vi "Big Boolean Cluster.vi"(1 "Cluster":T1) -> (0 "Cluster out":T1)   [LabVIEW 2010]
types:
  T1 = cluster{"Boolean":bool, "Boolean 2":bool, "Boolean 3":bool, "Boolean 4":bool, "Boolean 5":bool, "Boolean 6":bool, "Boolean 7":bool, "Boolean 8":bool, "Boolean 9":bool, "Boolean 10":bool, "Boolean 11":bool, "Boolean 12":bool, "Boolean 13":bool, "Boolean 14":bool, "Boolean 15":bool, "Boolean 16":bool, "Boolean 17":bool, "Boolean 18":bool, "Boolean 19":bool, "Boolean 20":bool, "Boolean 21":bool, "Boolean 22":bool, "Boolean 23":bool, "Boolean 24":bool, "Boolean 25":bool, "Boolean 26":bool, "Boolean 27":bool, "Boolean 28":bool, "Boolean 29":bool, "Boolean 30":bool, "Boolean 31":bool, "Boolean 32":bool, "Boolean 33":bool, "Boolean 34":bool, "Boolean 35":bool, "Boolean 36":bool, "Boolean 37":bool, "Boolean 38":bool, "Boolean 39":bool, "Boolean 40":bool, "Boolean 41":bool, "Boolean 42":bool, "Boolean 43":bool, "Boolean 44":bool, "Boolean 45":bool, "Boolean 46":bool, "Boolean 47":bool, "Boolean 48":bool, "Boolean 49":bool, "Boolean 50":bool, "Boolean 51":bool, "Boolean 52":bool, "Boolean 53":bool, "Boolean 54":bool, "Boolean 55":bool, "Boolean 56":bool, "Boolean 57":bool, "Boolean 58":bool, "Boolean 59":bool, "Boolean 60":bool, "Boolean 61":bool, "Boolean 62":bool, "Boolean 63":bool, "Boolean 64":bool, "Boolean 65":bool, "Boolean 66":bool, "Boolean 67":bool, "Boolean 68":bool, "Boolean 69":bool, "Boolean 70":bool, "Boolean 71":bool, "Boolean 72":bool, "Boolean 73":bool, "Boolean 74":bool, "Boolean 75":bool, "Boolean 76":bool, "Boolean 77":bool, "Boolean 78":bool, "Boolean 79":bool, "Boolean 80":bool, "Boolean 81":bool, "Boolean 82":bool, "Boolean 83":bool, "Boolean 84":bool, "Boolean 85":bool, "Boolean 86":bool, "Boolean 87":bool, "Boolean 88":bool, "Boolean 89":bool, "Boolean 90":bool, "Boolean 91":bool, "Boolean 92":bool, "Boolean 93":bool, "Boolean 94":bool, "Boolean 95":bool, "Boolean 96":bool, "Boolean 97":bool, "Boolean 98":bool, "Boolean 99":bool, "Boolean 100":bool, "Boolean 101":bool, "Boolean 102":bool, "Boolean 103":bool, "Boolean 104":bool, "Boolean 105":bool, "Boolean 106":bool, "Boolean 107":bool, "Boolean 108":bool, "Boolean 109":bool, "Boolean 110":bool, "Boolean 111":bool, "Boolean 112":bool, "Boolean 113":bool, "Boolean 114":bool, "Boolean 115":bool, "Boolean 116":bool, "Boolean 117":bool, "Boolean 118":bool, "Boolean 119":bool, "Boolean 120":bool, "Boolean 121":bool, "Boolean 122":bool, "Boolean 123":bool, "Boolean 124":bool, "Boolean 125":bool, "Boolean 126":bool, "Boolean 127":bool, "Boolean 128":bool, "Boolean 129":bool, "Boolean 130":bool, "Boolean 131":bool, "Boolean 132":bool, "Boolean 133":bool, "Boolean 134":bool, "Boolean 135":bool, "Boolean 136":bool, "Boolean 137":bool, "Boolean 138":bool, "Boolean 139":bool, "Boolean 140":bool, "Boolean 141":bool, "Boolean 142":bool, "Boolean 143":bool, "Boolean 144":bool, "Boolean 145":bool, "Boolean 146":bool, "Boolean 147":bool, "Boolean 148":bool, "Boolean 149":bool, "Boolean 150":bool, "Boolean 151":bool, "Boolean 152":bool, "Boolean 153":bool, "Boolean 154":bool, "Boolean 155":bool, "Boolean 156":bool, "Boolean 157":bool, "Boolean 158":bool, "Boolean 159":bool, "Boolean 160":bool, "Boolean 161":bool, "Boolean 162":bool, "Boolean 163":bool, "Boolean 164":bool, "Boolean 165":bool, "Boolean 166":bool, "Boolean 167":bool, "Boolean 168":bool, "Boolean 169":bool, "Boolean 170":bool, "Boolean 171":bool, "Boolean 172":bool, "Boolean 173":bool, "Boolean 174":bool, "Boolean 175":bool, "Boolean 176":bool, "Boolean 177":bool, "Boolean 178":bool, "Boolean 179":bool, "Boolean 180":bool, "Boolean 181":bool, "Boolean 182":bool, "Boolean 183":bool, "Boolean 184":bool, "Boolean 185":bool, "Boolean 186":bool, "Boolean 187":bool, "Boolean 188":bool, "Boolean 189":bool, "Boolean 190":bool, "Boolean 191":bool, "Boolean 192":bool, "Boolean 193":bool, "Boolean 194":bool, "Boolean 195":bool, "Boolean 196":bool, "Boolean 197":bool, "Boolean 198":bool, "Boolean 199":bool, "Boolean 200":bool, "Boolean 201":bool, "Boolean 202":bool, "Boolean 203":bool, "Boolean 204":bool, "Boolean 205":bool, "Boolean 206":bool, "Boolean 207":bool, "Boolean 208":bool, "Boolean 209":bool, "Boolean 210":bool, "Boolean 211":bool, "Boolean 212":bool, "Boolean 213":bool, "Boolean 214":bool, "Boolean 215":bool, "Boolean 216":bool, "Boolean 217":bool, "Boolean 218":bool, "Boolean 219":bool, "Boolean 220":bool, "Boolean 221":bool, "Boolean 222":bool, "Boolean 223":bool, "Boolean 224":bool, "Boolean 225":bool, "Boolean 226":bool, "Boolean 227":bool, "Boolean 228":bool, "Boolean 229":bool, "Boolean 230":bool, "Boolean 231":bool, "Boolean 232":bool, "Boolean 233":bool, "Boolean 234":bool, "Boolean 235":bool, "Boolean 236":bool, "Boolean 237":bool, "Boolean 238":bool, "Boolean 239":bool, "Boolean 240":bool, "Boolean 241":bool, "Boolean 242":bool, "Boolean 243":bool, "Boolean 244":bool, "Boolean 245":bool, "Boolean 246":bool, "Boolean 247":bool, "Boolean 248":bool, "Boolean 249":bool, "Boolean 250":bool, "Boolean 251":bool, "Boolean 252":bool, "Boolean 253":bool, "Boolean 254":bool, "Boolean 255":bool, "Boolean 256":bool, "Boolean 257":bool, "Boolean 258":bool, "Boolean 259":bool, "Boolean 260":bool, "Boolean 261":bool, "Boolean 262":bool, "Boolean 263":bool, "Boolean 264":bool, "Boolean 265":bool, "Boolean 266":bool, "Boolean 267":bool, "Boolean 268":bool, "Boolean 269":bool, "Boolean 270":bool, "Boolean 271":bool, "Boolean 272":bool, "Boolean 273":bool, "Boolean 274":bool, "Boolean 275":bool, "Boolean 276":bool, "Boolean 277":bool, "Boolean 278":bool, "Boolean 279":bool, "Boolean 280":bool, "Boolean 281":bool, "Boolean 282":bool, "Boolean 283":bool, "Boolean 284":bool, "Boolean 285":bool, "Boolean 286":bool, "Boolean 287":bool, "Boolean 288":bool, "Boolean 289":bool, "Boolean 290":bool, "Boolean 291":bool, "Boolean 292":bool, "Boolean 293":bool, "Boolean 294":bool, "Boolean 295":bool, "Boolean 296":bool, "Boolean 297":bool, "Boolean 298":bool, "Boolean 299":bool, "Boolean 300":bool, "Boolean 301":bool, "Boolean 302":bool, "Boolean 303":bool, "Boolean 304":bool, "Boolean 305":bool, "Boolean 306":bool, "Boolean 307":bool, "Boolean 308":bool, "Boolean 309":bool, "Boolean 310":bool, "Boolean 311":bool, "Boolean 312":bool, "Boolean 313":bool, "Boolean 314":bool, "Boolean 315":bool, "Boolean 316":bool, "Boolean 317":bool, "Boolean 318":bool, "Boolean 319":bool, "Boolean 320":bool, "Boolean 321":bool, "Boolean 322":bool, "Boolean 323":bool, "Boolean 324":bool, "Boolean 325":bool, "Boolean 326":bool, "Boolean 327":bool, "Boolean 328":bool, "Boolean 329":bool, "Boolean 330":bool, "Boolean 331":bool, "Boolean 332":bool, "Boolean 333":bool, "Boolean 334":bool, "Boolean 335":bool, "Boolean 336":bool, "Boolean 337":bool, "Boolean 338":bool, "Boolean 339":bool, "Boolean 340":bool, "Boolean 341":bool, "Boolean 342":bool, "Boolean 343":bool, "Boolean 344":bool, "Boolean 345":bool, "Boolean 346":bool, "Boolean 347":bool, "Boolean 348":bool, "Boolean 349":bool, "Boolean 350":bool, "Boolean 351":bool, "Boolean 352":bool, "Boolean 353":bool, "Boolean 354":bool, "Boolean 355":bool, "Boolean 356":bool, "Boolean 357":bool, "Boolean 358":bool, "Boolean 359":bool, "Boolean 360":bool, "Boolean 361":bool, "Boolean 362":bool, "Boolean 363":bool, "Boolean 364":bool, "Boolean 365":bool, "Boolean 366":bool, "Boolean 367":bool, "Boolean 368":bool, "Boolean 369":bool, "Boolean 370":bool, "Boolean 371":bool, "Boolean 372":bool, "Boolean 373":bool, "Boolean 374":bool, "Boolean 375":bool, "Boolean 376":bool, "Boolean 377":bool, "Boolean 378":bool, "Boolean 379":bool, "Boolean 380":bool, "Boolean 381":bool, "Boolean 382":bool, "Boolean 383":bool, "Boolean 384":bool, "Boolean 385":bool, "Boolean 386":bool, "Boolean 387":bool, "Boolean 388":bool, "Boolean 389":bool, "Boolean 390":bool, "Boolean 391":bool, "Boolean 392":bool, "Boolean 393":bool, "Boolean 394":bool, "Boolean 395":bool, "Boolean 396":bool, "Boolean 397":bool, "Boolean 398":bool, "Boolean 399":bool, "Boolean 400":bool, "Boolean 401":bool, "Boolean 402":bool, "Boolean 403":bool, "Boolean 404":bool, "Boolean 405":bool, "Boolean 406":bool, "Boolean 407":bool, "Boolean 408":bool, "Boolean 409":bool, "Boolean 410":bool, "Boolean 411":bool, "Boolean 412":bool, "Boolean 413":bool, "Boolean 414":bool, "Boolean 415":bool, "Boolean 416":bool, "Boolean 417":bool, "Boolean 418":bool, "Boolean 419":bool, "Boolean 420":bool, "Boolean 421":bool, "Boolean 422":bool, "Boolean 423":bool, "Boolean 424":bool, "Boolean 425":bool, "Boolean 426":bool, "Boolean 427":bool, "Boolean 428":bool, "Boolean 429":bool, "Boolean 430":bool, "Boolean 431":bool, "Boolean 432":bool, "Boolean 433":bool, "Boolean 434":bool, "Boolean 435":bool, "Boolean 436":bool, "Boolean 437":bool, "Boolean 438":bool, "Boolean 439":bool, "Boolean 440":bool, "Boolean 441":bool, "Boolean 442":bool, "Boolean 443":bool, "Boolean 444":bool, "Boolean 445":bool, "Boolean 446":bool, "Boolean 447":bool, "Boolean 448":bool, "Boolean 449":bool, "Boolean 450":bool, "Boolean 451":bool, "Boolean 452":bool, "Boolean 453":bool, "Boolean 454":bool, "Boolean 455":bool, "Boolean 456":bool, "Boolean 457":bool, "Boolean 458":bool, "Boolean 459":bool, "Boolean 460":bool, "Boolean 461":bool, "Boolean 462":bool, "Boolean 463":bool, "Boolean 464":bool, "Boolean 465":bool, "Boolean 466":bool, "Boolean 467":bool, "Boolean 468":bool, "Boolean 469":bool, "Boolean 470":bool, "Boolean 471":bool, "Boolean 472":bool, "Boolean 473":bool, "Boolean 474":bool, "Boolean 475":bool, "Boolean 476":bool, "Boolean 477":bool, "Boolean 478":bool, "Boolean 479":bool, "Boolean 480":bool, "Boolean 481":bool, "Boolean 482":bool, "Boolean 483":bool, "Boolean 484":bool, "Boolean 485":bool, "Boolean 486":bool, "Boolean 487":bool, "Boolean 488":bool, "Boolean 489":bool, "Boolean 490":bool, "Boolean 491":bool, "Boolean 492":bool, "Boolean 493":bool, "Boolean 494":bool, "Boolean 495":bool, "Boolean 496":bool, "Boolean 497":bool, "Boolean 498":bool, "Boolean 499":bool, "Boolean 500":bool, "Boolean 501":bool, "Boolean 502":bool, "Boolean 503":bool, "Boolean 504":bool, "Boolean 505":bool, "Boolean 506":bool, "Boolean 507":bool, "Boolean 508":bool, "Boolean 509":bool, "Boolean 510":bool, "Boolean 511":bool, "Boolean 512":bool, "Boolean 513":bool, "Boolean 514":bool, "Boolean 515":bool, "Boolean 516":bool, "Boolean 517":bool, "Boolean 518":bool, "Boolean 519":bool, "Boolean 520":bool, "Boolean 521":bool, "Boolean 522":bool, "Boolean 523":bool, "Boolean 524":bool, "Boolean 525":bool, "Boolean 526":bool, "Boolean 527":bool, "Boolean 528":bool, "Boolean 529":bool, "Boolean 530":bool, "Boolean 531":bool, "Boolean 532":bool, "Boolean 533":bool, "Boolean 534":bool, "Boolean 535":bool, "Boolean 536":bool, "Boolean 537":bool, "Boolean 538":bool, "Boolean 539":bool, "Boolean 540":bool, "Boolean 541":bool, "Boolean 542":bool, "Boolean 543":bool, "Boolean 544":bool, "Boolean 545":bool, "Boolean 546":bool, "Boolean 547":bool, "Boolean 548":bool, "Boolean 549":bool, "Boolean 550":bool, "Boolean 551":bool, "Boolean 552":bool, "Boolean 553":bool, "Boolean 554":bool, "Boolean 555":bool, "Boolean 556":bool, "Boolean 557":bool, "Boolean 558":bool, "Boolean 559":bool, "Boolean 560":bool, "Boolean 561":bool, "Boolean 562":bool, "Boolean 563":bool, "Boolean 564":bool, "Boolean 565":bool, "Boolean 566":bool, "Boolean 567":bool, "Boolean 568":bool, "Boolean 569":bool, "Boolean 570":bool, "Boolean 571":bool, "Boolean 572":bool, "Boolean 573":bool, "Boolean 574":bool, "Boolean 575":bool, "Boolean 576":bool, "Boolean 577":bool, "Boolean 578":bool, "Boolean 579":bool, "Boolean 580":bool, "Boolean 581":bool, "Boolean 582":bool, "Boolean 583":bool, "Boolean 584":bool, "Boolean 585":bool, "Boolean 586":bool, "Boolean 587":bool, "Boolean 588":bool, "Boolean 589":bool, "Boolean 590":bool, "Boolean 591":bool, "Boolean 592":bool, "Boolean 593":bool, "Boolean 594":bool, "Boolean 595":bool, "Boolean 596":bool, "Boolean 597":bool, "Boolean 598":bool, "Boolean 599":bool, "Boolean 600":bool, "Boolean 601":bool, "Boolean 602":bool, "Boolean 603":bool, "Boolean 604":bool, "Boolean 605":bool, "Boolean 606":bool, "Boolean 607":bool, "Boolean 608":bool, "Boolean 609":bool, "Boolean 610":bool, "Boolean 611":bool, "Boolean 612":bool, "Boolean 613":bool, "Boolean 614":bool, "Boolean 615":bool, "Boolean 616":bool, "Boolean 617":bool, "Boolean 618":bool, "Boolean 619":bool, "Boolean 620":bool, "Boolean 621":bool, "Boolean 622":bool, "Boolean 623":bool, "Boolean 624":bool, "Boolean 625":bool, "Boolean 626":bool, "Boolean 627":bool, "Boolean 628":bool, "Boolean 629":bool, "Boolean 630":bool, "Boolean 631":bool, "Boolean 632":bool, "Boolean 633":bool, "Boolean 634":bool, "Boolean 635":bool, "Boolean 636":bool, "Boolean 637":bool, "Boolean 638":bool, "Boolean 639":bool, "Boolean 640":bool, "Boolean 641":bool, "Boolean 642":bool, "Boolean 643":bool, "Boolean 644":bool, "Boolean 645":bool, "Boolean 646":bool, "Boolean 647":bool, "Boolean 648":bool, "Boolean 649":bool, "Boolean 650":bool, "Boolean 651":bool, "Boolean 652":bool, "Boolean 653":bool, "Boolean 654":bool, "Boolean 655":bool, "Boolean 656":bool, "Boolean 657":bool, "Boolean 658":bool, "Boolean 659":bool, "Boolean 660":bool, "Boolean 661":bool, "Boolean 662":bool, "Boolean 663":bool, "Boolean 664":bool, "Boolean 665":bool, "Boolean 666":bool, "Boolean 667":bool, "Boolean 668":bool, "Boolean 669":bool, "Boolean 670":bool, "Boolean 671":bool, "Boolean 672":bool, "Boolean 673":bool, "Boolean 674":bool, "Boolean 675":bool, "Boolean 676":bool, "Boolean 677":bool, "Boolean 678":bool, "Boolean 679":bool, "Boolean 680":bool, "Boolean 681":bool, "Boolean 682":bool, "Boolean 683":bool, "Boolean 684":bool, "Boolean 685":bool, "Boolean 686":bool, "Boolean 687":bool, "Boolean 688":bool, "Boolean 689":bool, "Boolean 690":bool, "Boolean 691":bool, "Boolean 692":bool, "Boolean 693":bool, "Boolean 694":bool, "Boolean 695":bool, "Boolean 696":bool, "Boolean 697":bool, "Boolean 698":bool, "Boolean 699":bool, "Boolean 700":bool, "Boolean 701":bool, "Boolean 702":bool, "Boolean 703":bool, "Boolean 704":bool, "Boolean 705":bool, "Boolean 706":bool, "Boolean 707":bool, "Boolean 708":bool, "Boolean 709":bool, "Boolean 710":bool, "Boolean 711":bool, "Boolean 712":bool, "Boolean 713":bool, "Boolean 714":bool, "Boolean 715":bool, "Boolean 716":bool, "Boolean 717":bool, "Boolean 718":bool, "Boolean 719":bool, "Boolean 720":bool, "Boolean 721":bool, "Boolean 722":bool, "Boolean 723":bool, "Boolean 724":bool, "Boolean 725":bool, "Boolean 726":bool, "Boolean 727":bool, "Boolean 728":bool, "Boolean 729":bool, "Boolean 730":bool, "Boolean 731":bool, "Boolean 732":bool, "Boolean 733":bool, "Boolean 734":bool, "Boolean 735":bool, "Boolean 736":bool, "Boolean 737":bool, "Boolean 738":bool, "Boolean 739":bool, "Boolean 740":bool, "Boolean 741":bool, "Boolean 742":bool, "Boolean 743":bool, "Boolean 744":bool, "Boolean 745":bool, "Boolean 746":bool, "Boolean 747":bool, "Boolean 748":bool, "Boolean 749":bool, "Boolean 750":bool, "Boolean 751":bool, "Boolean 752":bool, "Boolean 753":bool, "Boolean 754":bool, "Boolean 755":bool, "Boolean 756":bool, "Boolean 757":bool, "Boolean 758":bool, "Boolean 759":bool, "Boolean 760":bool, "Boolean 761":bool, "Boolean 762":bool, "Boolean 763":bool, "Boolean 764":bool, "Boolean 765":bool, "Boolean 766":bool, "Boolean 767":bool, "Boolean 768":bool, "Boolean 769":bool, "Boolean 770":bool, "Boolean 771":bool, "Boolean 772":bool, "Boolean 773":bool, "Boolean 774":bool, "Boolean 775":bool, "Boolean 776":bool, "Boolean 777":bool, "Boolean 778":bool, "Boolean 779":bool, "Boolean 780":bool, "Boolean 781":bool, "Boolean 782":bool, "Boolean 783":bool, "Boolean 784":bool, "Boolean 785":bool, "Boolean 786":bool, "Boolean 787":bool, "Boolean 788":bool, "Boolean 789":bool, "Boolean 790":bool, "Boolean 791":bool, "Boolean 792":bool, "Boolean 793":bool, "Boolean 794":bool, "Boolean 795":bool, "Boolean 796":bool, "Boolean 797":bool, "Boolean 798":bool, "Boolean 799":bool, "Boolean 800":bool, "Boolean 801":bool, "Boolean 802":bool, "Boolean 803":bool, "Boolean 804":bool, "Boolean 805":bool, "Boolean 806":bool, "Boolean 807":bool, "Boolean 808":bool, "Boolean 809":bool, "Boolean 810":bool, "Boolean 811":bool, "Boolean 812":bool, "Boolean 813":bool, "Boolean 814":bool, "Boolean 815":bool, "Boolean 816":bool, "Boolean 817":bool, "Boolean 818":bool, "Boolean 819":bool, "Boolean 820":bool, "Boolean 821":bool, "Boolean 822":bool, "Boolean 823":bool, "Boolean 824":bool, "Boolean 825":bool, "Boolean 826":bool, "Boolean 827":bool, "Boolean 828":bool, "Boolean 829":bool, "Boolean 830":bool, "Boolean 831":bool, "Boolean 832":bool, "Boolean 833":bool, "Boolean 834":bool, "Boolean 835":bool, "Boolean 836":bool, "Boolean 837":bool, "Boolean 838":bool, "Boolean 839":bool, "Boolean 840":bool, "Boolean 841":bool, "Boolean 842":bool, "Boolean 843":bool, "Boolean 844":bool, "Boolean 845":bool, "Boolean 846":bool, "Boolean 847":bool, "Boolean 848":bool, "Boolean 849":bool, "Boolean 850":bool, "Boolean 851":bool, "Boolean 852":bool, "Boolean 853":bool, "Boolean 854":bool, "Boolean 855":bool, "Boolean 856":bool, "Boolean 857":bool, "Boolean 858":bool, "Boolean 859":bool, "Boolean 860":bool, "Boolean 861":bool, "Boolean 862":bool, "Boolean 863":bool, "Boolean 864":bool, "Boolean 865":bool, "Boolean 866":bool, "Boolean 867":bool, "Boolean 868":bool, "Boolean 869":bool, "Boolean 870":bool, "Boolean 871":bool, "Boolean 872":bool, "Boolean 873":bool, "Boolean 874":bool, "Boolean 875":bool, "Boolean 876":bool, "Boolean 877":bool, "Boolean 878":bool, "Boolean 879":bool, "Boolean 880":bool, "Boolean 881":bool, "Boolean 882":bool, "Boolean 883":bool, "Boolean 884":bool, "Boolean 885":bool, "Boolean 886":bool, "Boolean 887":bool, "Boolean 888":bool, "Boolean 889":bool, "Boolean 890":bool, "Boolean 891":bool, "Boolean 892":bool, "Boolean 893":bool, "Boolean 894":bool, "Boolean 895":bool, "Boolean 896":bool, "Boolean 897":bool, "Boolean 898":bool, "Boolean 899":bool, "Boolean 900":bool, "Boolean 901":bool, "Boolean 902":bool, "Boolean 903":bool, "Boolean 904":bool, "Boolean 905":bool, "Boolean 906":bool, "Boolean 907":bool, "Boolean 908":bool, "Boolean 909":bool, "Boolean 910":bool, "Boolean 911":bool, "Boolean 912":bool, "Boolean 913":bool, "Boolean 914":bool, "Boolean 915":bool, "Boolean 916":bool, "Boolean 917":bool, "Boolean 918":bool, "Boolean 919":bool, "Boolean 920":bool, "Boolean 921":bool, "Boolean 922":bool, "Boolean 923":bool, "Boolean 924":bool, "Boolean 925":bool, "Boolean 926":bool, "Boolean 927":bool, "Boolean 928":bool, "Boolean 929":bool, "Boolean 930":bool, "Boolean 931":bool, "Boolean 932":bool, "Boolean 933":bool, "Boolean 934":bool, "Boolean 935":bool, "Boolean 936":bool, "Boolean 937":bool, "Boolean 938":bool, "Boolean 939":bool, "Boolean 940":bool, "Boolean 941":bool, "Boolean 942":bool, "Boolean 943":bool, "Boolean 944":bool, "Boolean 945":bool, "Boolean 946":bool, "Boolean 947":bool, "Boolean 948":bool, "Boolean 949":bool, "Boolean 950":bool, "Boolean 951":bool, "Boolean 952":bool, "Boolean 953":bool, "Boolean 954":bool, "Boolean 955":bool, "Boolean 956":bool, "Boolean 957":bool, "Boolean 958":bool, "Boolean 959":bool, "Boolean 960":bool, "Boolean 961":bool, "Boolean 962":bool, "Boolean 963":bool, "Boolean 964":bool, "Boolean 965":bool, "Boolean 966":bool, "Boolean 967":bool, "Boolean 968":bool, "Boolean 969":bool, "Boolean 970":bool, "Boolean 971":bool, "Boolean 972":bool, "Boolean 973":bool, "Boolean 974":bool, "Boolean 975":bool, "Boolean 976":bool, "Boolean 977":bool, "Boolean 978":bool, "Boolean 979":bool, "Boolean 980":bool, "Boolean 981":bool, "Boolean 982":bool, "Boolean 983":bool, "Boolean 984":bool, "Boolean 985":bool, "Boolean 986":bool, "Boolean 987":bool, "Boolean 988":bool, "Boolean 989":bool, "Boolean 990":bool, "Boolean 991":bool, "Boolean 992":bool, "Boolean 993":bool, "Boolean 994":bool, "Boolean 995":bool, "Boolean 996":bool, "Boolean 997":bool, "Boolean 998":bool, "Boolean 999":bool, "Boolean 1000":bool}
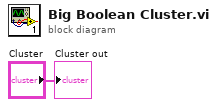
[diagram p0: block diagram]
diagram:
  "Cluster out" <- "Cluster"
